vi "Create Delimitted Data Line.vi"() -> ()   [LabVIEW 2018]
panel:
  out "Delimitted Line":string
  in  "delimitter (\\t)":string
  in  "Array":dbl[](array[numeric])
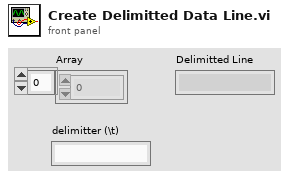
[diagram p1: front panel]
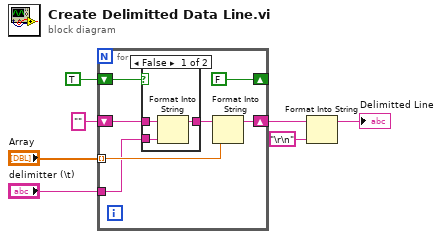
[diagram p0: block diagram]
diagram:
  n1 = for {
    tunnel: "Array" -> [w14] mode=indexing
    shift-right: [w8] -> w3
    shift-left: "" -> [w12]
    shift-right: [FALSE] -> _
    shift-left: TRUE -> [w9]
    tunnel: "delimitter (\\t)" -> [w10]
    n2 = case shown="False" w9 {
      tunnel: w12 -> [w17 w18]
      tunnel: [w16 w18] -> w11
      tunnel: w10 -> [w15 _]
      frame False {
        n3 = Format Into String(initial string=w17, w15) -> (resulting string=w16:string)  [unwired: 2 in, 1 out]
      }
      frame True {
      }
    }
    n4 = Format Into String(initial string=w11, w14) -> (resulting string=w8:string)  [unwired: 2 in, 1 out]
  }
  n5 = Format Into String(initial string=w3, "\r\n") -> (resulting string=→"Delimitted Line":string)  [unwired: 2 in, 1 out]
